vi "Fetch Room Details.vi"(0 "File Data Manager in":refnum<class "File Data Manager.lvclass">, 5 "Room No":string, 11 "error in (no error)":errorcluster) -> (4 "File Data Manager out":refnum<class "File Data Manager.lvclass">, 6 "Room Details":T1, 15 "error out":errorcluster)   [LabVIEW 2023, in "File Data Manager.lvlib" / "File Data Manager.lvclass"]
uses:
  File Data Manager.lvclass
  File Data Manager.lvclass/File Data Manager.ctl
  Central Data Manager/Central Data Manager/Central Data Manager.lvclass
  Central Data Manager/Central Data Manager/Room Occupancy Status.ctl
  Central Data Manager/Central Data Manager/Guest Details.ctl
  Central Data Manager/Central Data Manager/Room Details.ctl
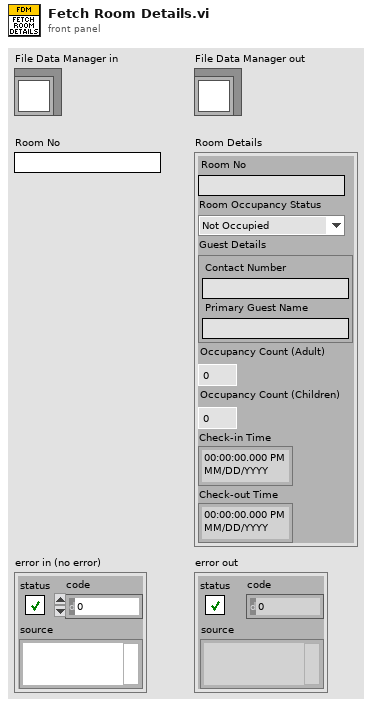
[diagram p1: front panel]
types:
  T1 = typedef "Central Data Manager.lvlib/Central Data Manager.lvclass/Room Details.ctl" = cluster{"Room No":string, "Room Occupancy Status":T2, "Guest Details":T3, "Occupancy Count (Adult)":dbl, "Occupancy Count (Children)":dbl, "Check-in Time":timestamp, "Check-out Time":timestamp}
  T2 = typedef "Central Data Manager.lvlib/Central Data Manager.lvclass/Room Occupancy Status.ctl" = enum16{"Not Occupied", "Occupied", "Under Maintainance", "Not Servicable"}
  T3 = typedef "Central Data Manager.lvlib/Central Data Manager.lvclass/Guest Details.ctl" = cluster{"Contact Number":string, "Primary Guest Name":string}
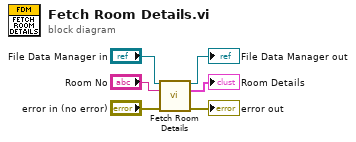
[diagram p0: block diagram]
diagram:
  n1 = call-parent "Fetch Room Details.vi"("Central Data Manager in"="File Data Manager in", "Room No"="Room No", "error in (no error)"="error in (no error)") -> ("Central Data Manager out"=→"File Data Manager out":refnum<class "File Data Manager.lvclass">, "Room Details"=→"Room Details":T1, "error out"=→"error out":errorcluster)  [unwired: 10 in]
